vi "高锰酸钾-ORP滴定曲线(子VI).vi"   [LabVIEW 2016, in "斯坦道CODMn.lvlib"]
uses:
  <vilib>/ptbypt/NI_PtbyPt.lvlib
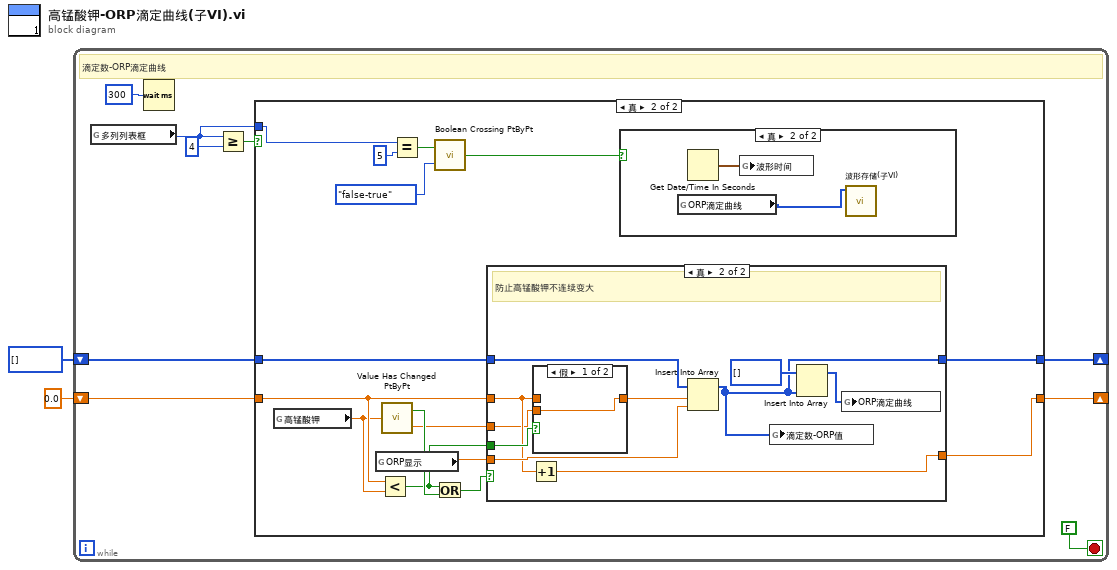
[diagram p0: block diagram]
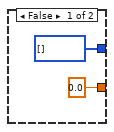
[diagram p2: hidden frame]
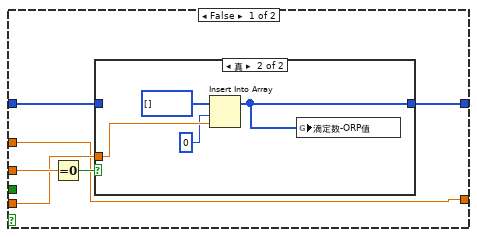
[diagram p4: hidden frame]
diagram:
  n1 = while {
    shift-right: [w8] -> _
    shift-left: u16[] [] ("ORP滴定曲线") -> [w9]
    shift-right: [w4] -> _
    shift-left: 0.0 -> [w5]
    stop <- FALSE stop-if-true
    # "滴定数-ORP滴定曲线"
    n2 = global read "运行时序全局变量.vi" "多列列表框"() -> (w3:i32)
    n3 = Wait (ms)(milliseconds to wait=u32 300 ("等待时间（毫秒）")) -> ()  [unwired: 1 out]
    n4 = Greater Or Equal?(x=w3, y=4) -> (x >= y?=w6:bool)
    n5 = case shown="真" w6 {
      tunnel: w9 -> [_ w28]
      tunnel: [u16[] [] ("ORP滴定曲线") w27] -> w8
      tunnel: w5 -> [_ w19]
      tunnel: [0.0 w18] -> w4
      tunnel: w3 -> [_ w16]
      frame False {
      }
      frame True {
        n6 = global read "COD内部交互全局.vi" "高锰酸钾"() -> (w15:dbl)
        n7 = global read "COD内部交互全局.vi" "ORP显示"() -> (w14:dbl)
        n8 = Less?(x=w19, y=w15) -> (x < y?=w17:bool)
        n9 = call <vilib>:"Value Has Changed PtByPt.vi"("input data point"=w15) -> ("has changed"=w26:bool, "output data point"=w25:dbl)  [unwired: 1 in]
        n10 = Equal?(x=w16, y=5) -> (x = y?=w23:bool)
        n11 = call <vilib>:"Boolean Crossing PtByPt.vi"("direction"=enum16{"either", "false-true", "true-false"}."false-true", "input"=w23) -> ("crossing"=w21:bool)  [unwired: 1 in]
        n12 = Or(x=w17, y=w26) -> (x .or. y?=w20:bool)
        n13 = case shown="真" w20 {
          tunnel: w28 -> [w35 w50]
          tunnel: [w34 w42] -> w27
          tunnel: w25 -> [w36 w44]
          tunnel: w14 -> [w32 w49]
          tunnel: w19 -> [w31 w46]
          tunnel: [w31 w48] -> w18
          tunnel: w17 -> [_ w47]
          frame False {
            n14 = Equal To 0?(x=w36) -> (x = 0?=w33:bool)
            n15 = case shown="真" w33 {
              tunnel: [w37 w38] -> w34
              tunnel: w35 -> [w37 _]
              tunnel: w32 -> [_ w40]
              frame False {
              }
              frame True {
                n16 = Insert Into Array(array=u16[] [] ("ORP滴定曲线"), index=0 ("索引"), new element=w40) -> (w38:u16[])
                n17 = global write "COD内部交互全局.vi" "滴定数-ORP值"(w38) -> ()
              }
            }
          }
          frame True {
            # "防止高锰酸钾不连续变大"
            n18 = Increment(x=w46) -> (x+1=w48:dbl)
            n19 = case shown="假" w47 {
              tunnel: w46 -> [_ w53]
              tunnel: [w52 w53] -> w45
              tunnel: w44 -> [w52 _]
              frame False {
              }
              frame True {
              }
            }
            n20 = Insert Into Array(array=w50, index=w45, new element=w49) -> (w42:u16[])
            n21 = global write "COD内部交互全局.vi" "滴定数-ORP值"(w42) -> ()
            n22 = Insert Into Array(array=u16[] [] ("ORP滴定曲线"), new element=w42) -> (w43:u16[])  [unwired: 1 in]
            n23 = global write "COD内部交互全局.vi" "ORP滴定曲线"(w43) -> ()
          }
        }
        n24 = case shown="真" w21 {
          frame False {
          }
          frame True {
            n25 = global read "COD内部交互全局.vi" "ORP滴定曲线"() -> (w29:u16[])
            n26 = Get Date/Time In Seconds() -> (seconds since 1Jan1904=w30:timestamp)
            n27 = global write "COD内部交互全局.vi" "波形时间"(w30) -> ()
            n28 = call "波形存储(子VI).vi"("ORP滴定曲线"=w29) -> ()  [unwired: 11 in]
          }
        }
      }
    }
  }
